vi "Close.vi"(8 "Error In":errorcluster, 11 "reference in":refnum<class "DBC Communicator.lvclass">) -> (0 "Error Out":errorcluster, 3 "reference out":refnum<class "DBC Communicator.lvclass">)   [LabVIEW 2025, in "DBC Communicator.lvclass"]
uses:
  DBC Communicator.lvclass
  Communicator/Communicator.lvclass
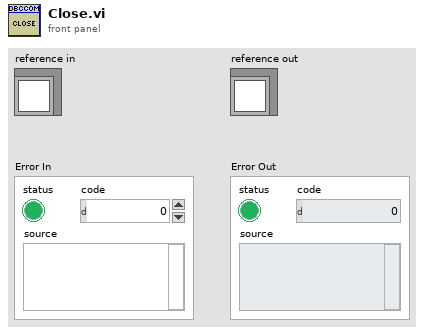
[diagram p1: front panel]
types:
  T1 = typedef "DBC Communicator.lvclass/ObjectAttributes.ctl" = cluster{"XNET Conversion Session":refnum<k21>, "Frame ID - Timestamp":map{u32, timestamp}, "Signals":cluster{"Names":string[], "Frame IDs":u32[]}}
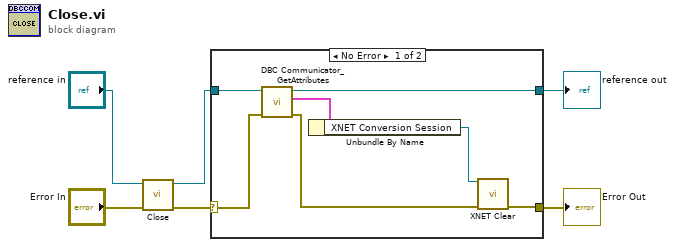
[diagram p0: block diagram]
diagram:
  n1 = call-parent "Close.vi"("Error In"="Error In", "Communicator in"="reference in") -> ("Error Out"=w3:errorcluster, "Communicator out"=w1:refnum<class "DBC Communicator.lvclass">)  [unwired: 8 in]
  n2 = case shown="No Error" w3 {
    selector: w3 -> [w7 w15]
    tunnel: [w10 w15] -> w5
    tunnel: [w12 w14] -> w4
    tunnel: w1 -> [w8 w14]
    frame No Error {
      n3 = call "DBC Communicator_GetAttributes.vi"("Error In"=w7, "reference in"=w8) -> ("Error Out"=w9:errorcluster, "Data"=w13:T1, "reference out"=w12:refnum<class "DBC Communicator.lvclass">)  [unwired: 6 in, 1 out]
      n4 = Unbundle By Name(w13) -> ("XNET Conversion Session"=w11:refnum<k21>)
      n5 = call <vilib>:"XNET Clear.vi"("session in"=w11, "error in (no error)"=w9) -> ("error out"=w10:errorcluster)  [unwired: 13 in]
    }
    frame Error {
    }
  }
  "Error Out" <- w5
  "reference out" <- w4
